vi "Spreadsheet Storage[OpenWriteClose] backslash.vi"() -> ()   [LabVIEW 2015]
panel:
  in  "Waveform Parameters":T1
  in  "Digitizing Parameters":T2
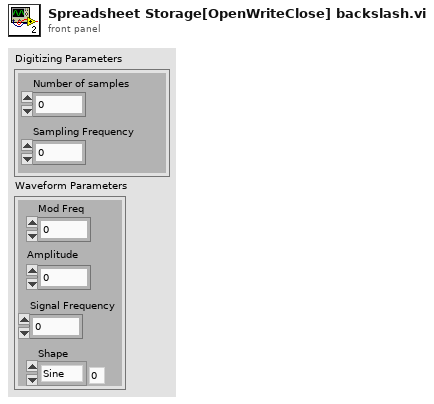
[diagram p1: front panel]
types:
  T1 = cluster{"Mod Freq":dbl, "Amplitude":dbl, "Shape":enum16{"Sine", "Cosine", "DC Level", "Square", "User Defined"}, "Signal Frequency":dbl}
  T2 = cluster{"Number of samples":dbl, "Sampling Frequency":dbl}
  T3 = enum16{"open", "replace", "create", "open or create", "replace or create", "replace or create with confirmation"}
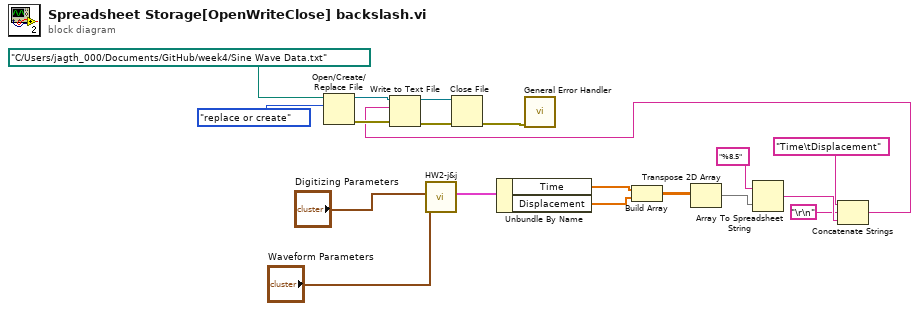
[diagram p0: block diagram]
diagram:
  n1 = Open/Create/Replace File(file path (use dialog)=path "C:/Users/jagth_000/Documents/GitHub/week4/Sine Wave Data.txt", operation (0:open)=T3."replace or create") -> (refnum out=w13:refnum<file>, error out=w11:errorcluster)  [unwired: 4 in, 1 out]
  n2 = call "HW2-j&j.vi"("AM Wave Parameters"="Waveform Parameters", "Digitizing Parameters"="Digitizing Parameters") -> ("AM Wave"=w17:cluster{"Time":dbl[], "Displacement":dbl[]})  [unwired: 9 in]
  n3 = Unbundle By Name(w17) -> ("Time"=w16:dbl[], "Displacement"=w15:dbl[])
  n4 = Build Array(w16, w15) -> (w7:dbl[][])
  n5 = Transpose 2D Array(2D array=w7) -> (transposed array=w5:dbl[][])
  n6 = Array To Spreadsheet String(array=w5, 3:"%8.5" ("format string")) -> (spreadsheet string=w4:string)  [unwired: 1 in]
  n7 = Concatenate Strings("Time\tDisplacement" ("string"), "\r\n", w4) -> (w1:string)
  n8 = Write to Text File(file (use dialog)=w13, text=w1, error in=w11) -> (refnum out=w12:refnum<file>, error out=w10:errorcluster)  [unwired: 1 in, 1 out]
  n9 = Close File(refnum=w12, error in=w10) -> (error out=w9:errorcluster)  [unwired: 1 out]
  n10 = call <vilib>:"General Error Handler.vi"("error in (no error)"=w9) -> ()  [unwired: 10 in, 5 out]
